vi "Read Loop Structure.vi"(8 "error in (no error)":errorcluster, 11 "Loop in":refnum<class "Loop.lvclass">) -> (0 "error out":errorcluster, 2 "Loop Structure":refnum<vi>, 3 "Loop out":refnum<class "Loop.lvclass">)   [LabVIEW 2015, in "Loop.lvclass"]
uses:
  Loop.lvclass
  Loop.lvclass/Loop.ctl
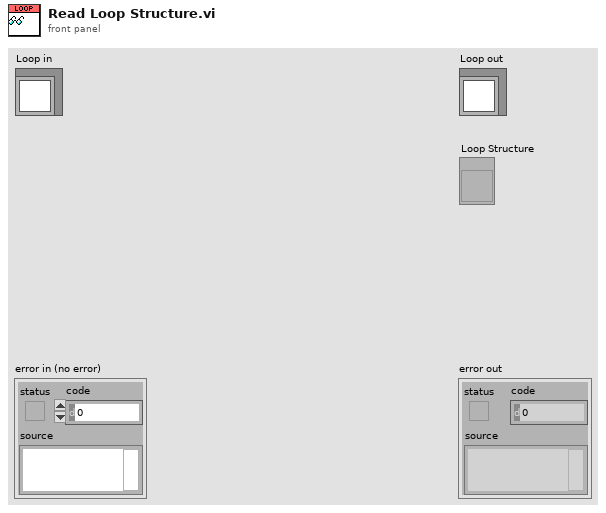
[diagram p1: front panel]
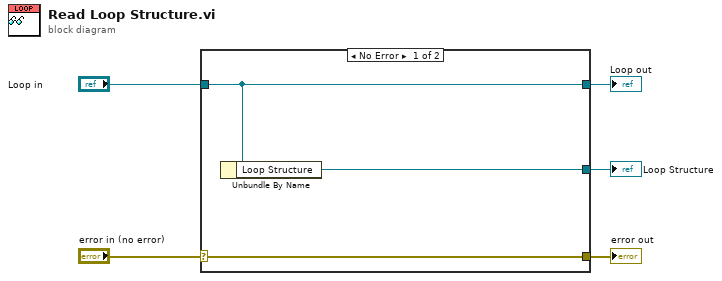
[diagram p0: block diagram]
diagram:
  n1 = case shown="No Error" "error in (no error)" {
    selector: "error in (no error)" -> [w8 w9]
    tunnel: [w8 w9] -> w4
    tunnel: [w7 w10] -> w2
    tunnel: "Loop in" -> [w7 w10]
    tunnel: [w6 _] -> w1
    frame No Error {
      n2 = Unbundle By Name(w7) -> ("Loop Structure"=w6:refnum<vi>)
    }
    frame Error {
    }
  }
  "error out" <- w4
  "Loop out" <- w2
  "Loop Structure" <- w1
